vi "Z Aux Trans Stringto Float.vi"(8 "error in (no error)":errorcluster caption="错误输入（无错误）", 9 "pfvlaue":sgl[](array[numeric])=array[4097 elements], 10 "inumes":i32, 11 "pstringin":string) -> (0 "error out":errorcluster caption="错误输出", 1 "pfvlaue out":sgl[](array[numeric]), 3 "function return":i32)   [LabVIEW 2015, in "zauxdll.lvlib"]
doc: "int32 __stdcall ZAux_TransStringtoFloat(const char* pstringin, int inumes, float pfvlaue[]);"
uses:
  zauxdll.lvlib
  Radar - 2015 32bit_autoqueue_angle_0319/zauxdll-2014/zauxdll.dll
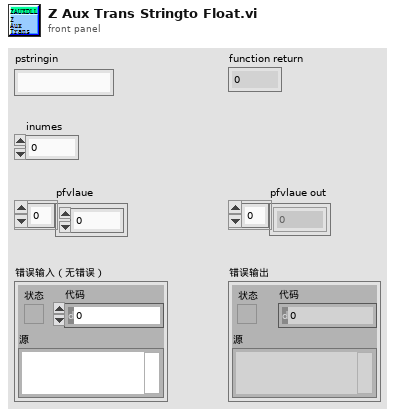
[diagram p1: front panel]
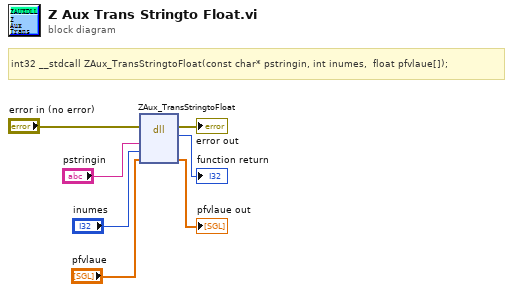
[diagram p0: block diagram]
diagram:
  # "int32 __stdcall ZAux_TransStringtoFloat(const char* pstringin, int inumes,  float pfvlaue[]);"
  n1 = dll-call lib="D:/vicomm case/cub/0717/Radar - 2015 32bit_autoqueue_angle_0319/zauxdll-2014/zauxdll.*" fn="ZAux_TransStringtoFloat"(error in="error in (no error)", "pstringin"="pstringin", "inumes"="inumes", "pfvlaue"="pfvlaue") -> (error out=→"error out":errorcluster, →"function return":i32, "pfvlaue"=→"pfvlaue out":sgl[])  [unwired: 4 in, 1 out]
